vi "op_biti_l0.vi"() -> ()   [LabVIEW 2009]
uses:
  <vilib>/Platform/portaccess.llb/Out Port8.vi
panel:
  out "Meter":dbl(knob) scale=0.0..3.0
  in  "Selector":u8(slide) scale=0.0..6.0
  out "Array":bool[](array[boolean])=[TRUE, FALSE, TRUE, FALSE, TRUE, FALSE, TRUE, FALSE]
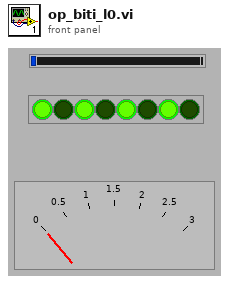
[diagram p1: front panel]
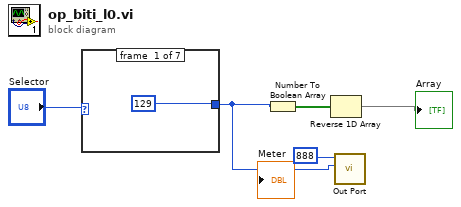
[diagram p0: block diagram]
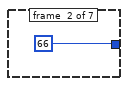
[diagram p2: hidden frame]
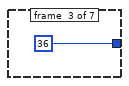
[diagram p3: hidden frame]
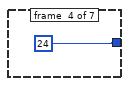
[diagram p4: hidden frame]
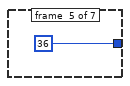
[diagram p5: hidden frame]
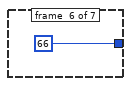
[diagram p6: hidden frame]
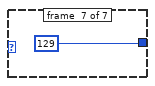
[diagram p7: hidden frame]
diagram:
  n1 = case shown="0, Default" "Selector" {
    tunnel: [u8 129 u8 66 u8 36 u8 24 u8 36 u8 66 u8 129] -> w1
    frame #0 {
    }
    frame #1 {
    }
    frame #2 {
    }
    frame #3 {
    }
    frame #4 {
    }
    frame #5 {
    }
    frame #6 {
    }
  }
  n2 = Number To Boolean Array(number=w1) -> (Boolean array=w5:bool[])
  n3 = Reverse 1D Array(array=w5) -> (reversed array=→"Array":bool[])
  n4 = call-poly <vilib>:"Out Port.vi"("write value"=w1, "address"=888) -> ()  [unwired: 7 in, 1 out]
